vi "Top Level FPGA.vi"   [LabVIEW 2014]
uses:
  <vilib>/rvi/DataTransferAndStorage/Container/XNode/niFpgaContainer.xnode
  <vilib>/Platform/TimedLoop/XDataNode/wakeup.ctl
  <vilib>/Platform/TimedLoop/XDataNode/XDNodeRunTimeDep.lvlib
  <vilib>/Platform/TimedLoop/XDataNode/nitl_modes.ctl
  <vilib>/Platform/TimedLoop/XDataNode/timing_clust.ctl
  <vilib>/Platform/TimedLoop/XDataNode/XDataNode.xnode
  <vilib>/eio/EIOMethodNode/EIOMethodNode.xnode
  <vilib>/rvi/eio/common/nirviEmuTemplateMethod_errors.vi
  <vilib>/rvi/FIFO/Fifo_Resource/nirvififoEmulationWrite.vi
  <vilib>/rvi/Memory/Memory_Emulation/nirvimemoryEmulation.vi
  <vilib>/rvi/Memory/Memory_Emulation/nirvimemoryFastEmulation.vi
  <vilib>/rvi/FIFO/Fifo_Resource/nirvififoEmulationRead.vi
types:
  T1 = typedef "XDNodeRunTimeDep.lvlib/timing_clust.ctl" = cluster{"Expected End [f-1]":u64, "Actual End [f-1]":u64, "Finished Late? [f-1]":bool, "Expected End [i-1]":u64, "Actual End [i-1]":u64, "Finished Late? [i-1]":bool, "Expected Start [i]":u64, "Actual Start [i]":u64, "Expected Start [f]":u64, "Actual Start [f]":u64, "Source Name":string, "Structure Name":string, "Period":i64, "Deadline":i64, "Offset":i64, "Start":i64, "Priority":i32, "Timeout":i32, "Mode":T2, "Wakeup Reason":T3, "Error":errorcluster, "Source Type":string, "Secondary Source Type":string, "Global End Time":u64, "Global Start Time":u64, "Frame Duration":u64, "Iteration Duration":u64, "Assigned CPU":i32, "I/O Scan Engine Mode":u32}
  T2 = typedef "XDNodeRunTimeDep.lvlib/nitl_modes.ctl" = enum32{"No Change", "Process missed periods, maintain original phase", "Discard missed periods, maintain original phase", "Process missed periods, ignore original phase", "Discard missed periods, ignore original phase"}
  T3 = typedef "XDNodeRunTimeDep.lvlib/wakeup.ctl" = enum32{"Normal", "Aborted", "Asynchronous wakeup", "Timing source error", "Timed loop error", "Timeout"}
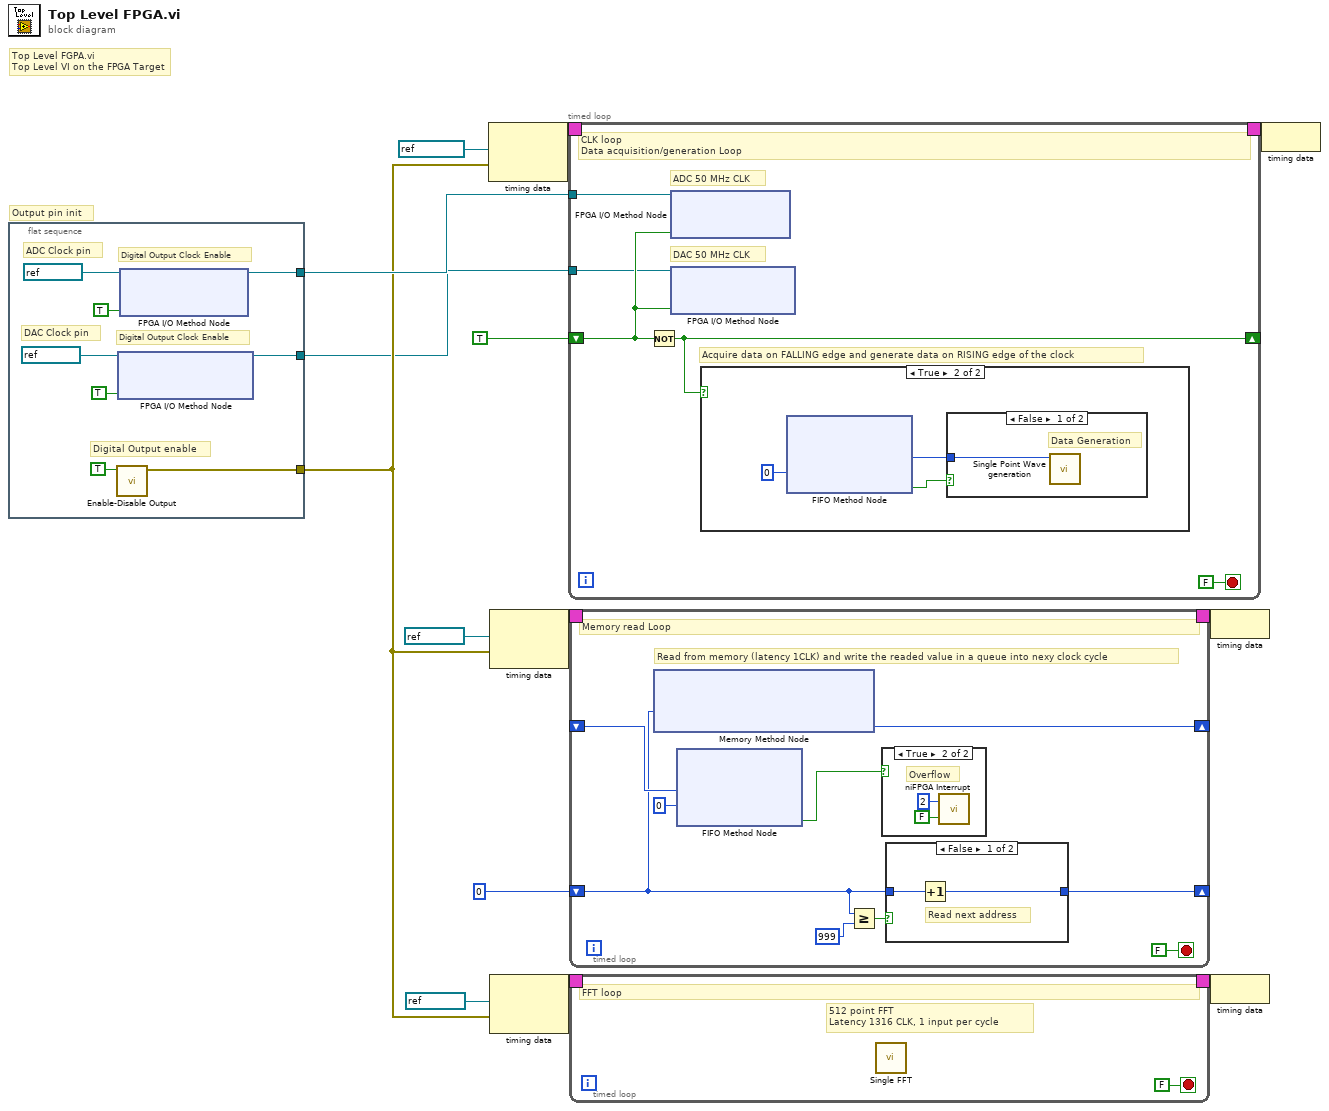
[diagram p0: block diagram]
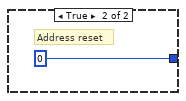
[diagram p3: hidden frame]
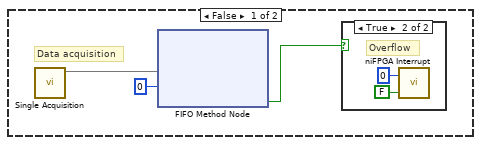
[diagram p4: hidden frame]
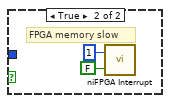
[diagram p6: hidden frame]
diagram:
  # "Output pin init"
  # "Top Level FGPA.vi\nTop Level VI on the FPGA Target"
  n1 = flat-sequence {
    tunnel: [w20] -> w6
    tunnel: [w18] -> w3
    tunnel: [w15] -> w1
    frame #0 {
      # "Digital Output Clock Enable"
      # "DAC Clock pin"
      # "Digital Output Clock Enable"
      # "Digital Output enable"
      # "ADC Clock pin"
      n2 = call "Enable-Disable Output.vi"("Enable"=TRUE) -> ("error out"=w18:errorcluster)  [unwired: 10 in]
      n3 = xnode "FPGA I/O Method Node"("FPGA I/O In"=refnum<k21> "DIO16", "Enable"=TRUE) -> ("FPGA I/O Out"=w15:refnum<k21>)
      n4 = xnode "FPGA I/O Method Node"("FPGA I/O In"=refnum<k21> "DIO17", "Enable"=TRUE) -> ("FPGA I/O Out"=w20:refnum<k21>)
    }
  }
  n5 = node-c288(refnum<k21> "100MHz" ("Source Name"), w3) -> (w14:T1)
  n6 = node-c288(refnum<k21> "50MHz" ("Source Name"), w3) -> (w12:T1)
  n7 = node-c288(refnum<k21> "50MHz" ("Source Name"), w3) -> (w10:T1)
  n8 = timed-loop {
    timing: w14 -> [_]
    timing-out: [_] -> w13
    shift-right: [w25] -> _
    shift-left: TRUE -> [w24]
    tunnel: w6 -> [w27]
    tunnel: w1 -> [w23]
    stop <- FALSE stop-if-true
    # "DAC 50 MHz CLK"
    # "Acquire data on FALLING edge and generate data on RISING edge of the clock"
    # "ADC 50 MHz CLK"
    # "CLK loop\nData acquisition/generation Loop"
    n9 = Not(x=w24) -> (.not. x?=w25:bool)
    n10 = xnode "FPGA I/O Method Node"("FPGA I/O In"=w27, "Data"=w24) -> ()  [unwired: 1 out]
    n11 = xnode "FPGA I/O Method Node"("FPGA I/O In"=w23, "Data"=w24) -> ()  [unwired: 1 out]
    n12 = case shown="True" w25 {
      frame False {
        # "Data acquisition"
        n13 = call "Single Acquisition.vi"() -> (3:w30)  [unwired: 9 in, 2 out]
        n14 = xnode ("FIFO Method Node")("Element"=w30, "Timeout"=0) -> ("Timed Out?"=w28:bool)  [unwired: 1 in, 1 out]
        n15 = case shown="True" w28 {
          frame False {
            # "Normal \nexecution"
          }
          frame True {
            # "Overflow"
            n16 = call <vilib>:"niFPGA Interrupt.vi"("Wait Until Cleared (F)"=FALSE, "IRQ Number (0)"=u8 0) -> ()  [unwired: 1 in]
          }
        }
      }
      frame True {
        n17 = xnode ("FIFO Method Node")("Timeout"=0) -> ("Element"=w35:i16, "Timed Out?"=w33:bool)  [unwired: 1 in, 1 out]
        n18 = case shown="False" w33 {
          tunnel: w35 -> [w36 _]
          frame False {
            # "Data Generation"
            n19 = call "Single Point Wave generation.vi"("Data To Write"=w36) -> ()  [unwired: 10 in, 1 out]
          }
          frame True {
            # "FPGA memory slow"
            n20 = call <vilib>:"niFPGA Interrupt.vi"("Wait Until Cleared (F)"=FALSE, "IRQ Number (0)"=u8 1) -> ()  [unwired: 1 in]
          }
        }
      }
    }
  }
  n21 = timed-loop {
    timing: w12 -> [_]
    timing-out: [_] -> w11
    shift-right: [w49] -> _
    shift-left: _ -> [w45]
    shift-right: [w46] -> _
    shift-left: u32 0 -> [w42]
    stop <- FALSE stop-if-true
    # "Read from memory (latency 1CLK) and write the readed value in a queue into nexy clock cycle"
    # "Memory read Loop"
    n22 = xnode ("Memory Method Node")("Address"=w42) -> ("Data"=w49:i16)  [unwired: 1 in, 1 out]
    n23 = xnode ("FIFO Method Node")("Element"=w45, "Timeout"=0) -> ("Timed Out?"=w41:bool)  [unwired: 1 in, 1 out]
    n24 = Greater Or Equal?(x=w42, y=u32 999) -> (x >= y?=w47:bool)
    n25 = case shown="True" w41 {
      frame False {
        # "Normal \nexecution"
      }
      frame True {
        # "Overflow"
        n26 = call <vilib>:"niFPGA Interrupt.vi"("Wait Until Cleared (F)"=FALSE, "IRQ Number (0)"=u8 2) -> ()  [unwired: 1 in]
      }
    }
    n27 = case shown="False" w47 {
      tunnel: w42 -> [w53 _]
      tunnel: [w52 u32 0] -> w46
      frame False {
        # "Read next address"
        n28 = Increment(x=w53) -> (x+1=w52:u32)
      }
      frame True {
        # "Address reset"
      }
    }
  }
  n29 = timed-loop {
    timing: w10 -> [_]
    timing-out: [_] -> w9
    stop <- FALSE stop-if-true
    # "512 point FFT \nLatency 1316 CLK, 1 input per cycle"
    # "FFT loop"
    n30 = call "Single FFT.vi"() -> ()  [unwired: 12 in]
  }
  n31 = node-c288(w11) -> ()
  n32 = node-c288(w9) -> ()
  n33 = node-c288(w13) -> ()
